vi "boolean type def tester.vi"() -> ()   [LabVIEW 2017]
uses:
  User Interface/Typedefs/Laser 1 switch.ctl
panel:
  in  "Boolean 2":bool=TRUE
  in  "stop":bool
  in  "Boolean":bool=TRUE
  out "Ls1 Status Ind":T1
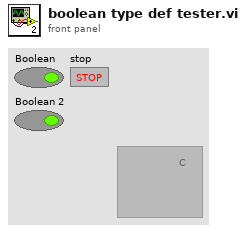
[diagram p1: front panel]
types:
  T1 = typedef "Laser 1 switch.ctl" = bool
  T2 = enum8{"Enabled", "Disabled", "Disabled and Grayed Out"}
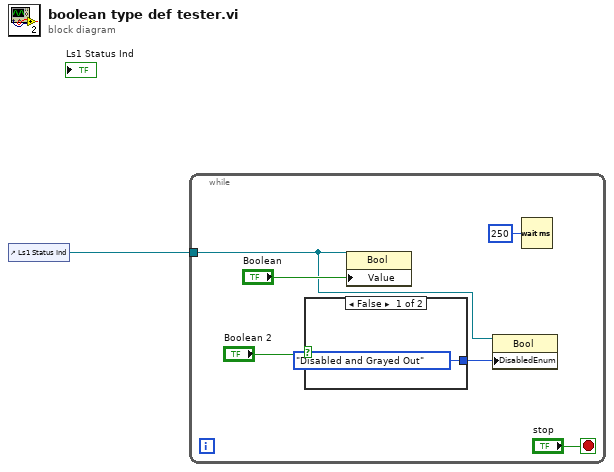
[diagram p0: block diagram]
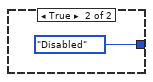
[diagram p2: hidden frame]
diagram:
  n1 = control-ref of="Ls1 Status Ind"() -> (w1:refnum<vi>)
  n2 = while {
    tunnel: w1 -> [w3]
    stop <- "stop" stop-if-true
    n3 = case shown="False" "Boolean 2" {
      tunnel: [T2."Disabled and Grayed Out" ("Disabled") T2."Disabled" ("Disabled")] -> w2
      frame False {
      }
      frame True {
      }
    }
    n4 = property class="Bool"(reference=w3, "Value"="Boolean") -> ()  [unwired: 1 in, 2 out]
    n5 = property class="Bool"(reference=w3, "DisabledEnum"=w2) -> ()  [unwired: 1 in, 2 out]
    n6 = Wait (ms)(milliseconds to wait=u32 250) -> ()  [unwired: 1 out]
  }
